vi "Update Set Temp.vi"(8 "error in (no error)":errorcluster, 9 "Setpoint":dbl, 10 "Run":bool, 11 "Test in":refnum<class "Test.lvclass">) -> (0 "error out":errorcluster, 3 "Test out":refnum<class "Test.lvclass">)   [LabVIEW 2019, in "Test.lvlib" / "Test.lvclass"]
uses:
  Test.lvclass
  Test.lvclass/Test.ctl
  <userlib>/_MGI/Application Control/MGI Get Value/MGI Get Value (String).vi
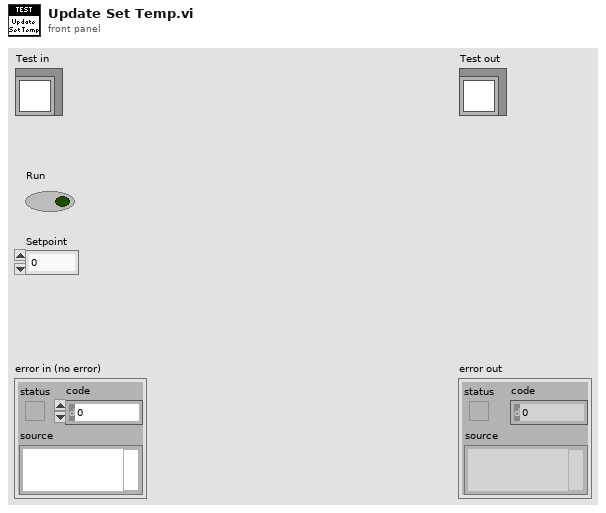
[diagram p1: front panel]
types:
  T1 = map{string, cluster{"Selected Heads":string, "Instrument":refnum<class "Message Enqueuer.lvclass">, "Platform":refnum<class "Message Enqueuer.lvclass">}}
  T2 = typedef "Test.lvlib/Cobra Data.ctl" = cluster{"M2 Dataset":cluster{"Read Temp":dbl, "Feedback":u8, "Set Temp":dbl}, "M1 Dataset":cluster{"Read Temp":dbl, "Feedback":u8, "Set Temp":dbl}, "Comp":bool}
  T3 = cluster{"Selected Heads":string, "Instrument":refnum<class "Message Enqueuer.lvclass">, "Platform":refnum<class "Message Enqueuer.lvclass">}
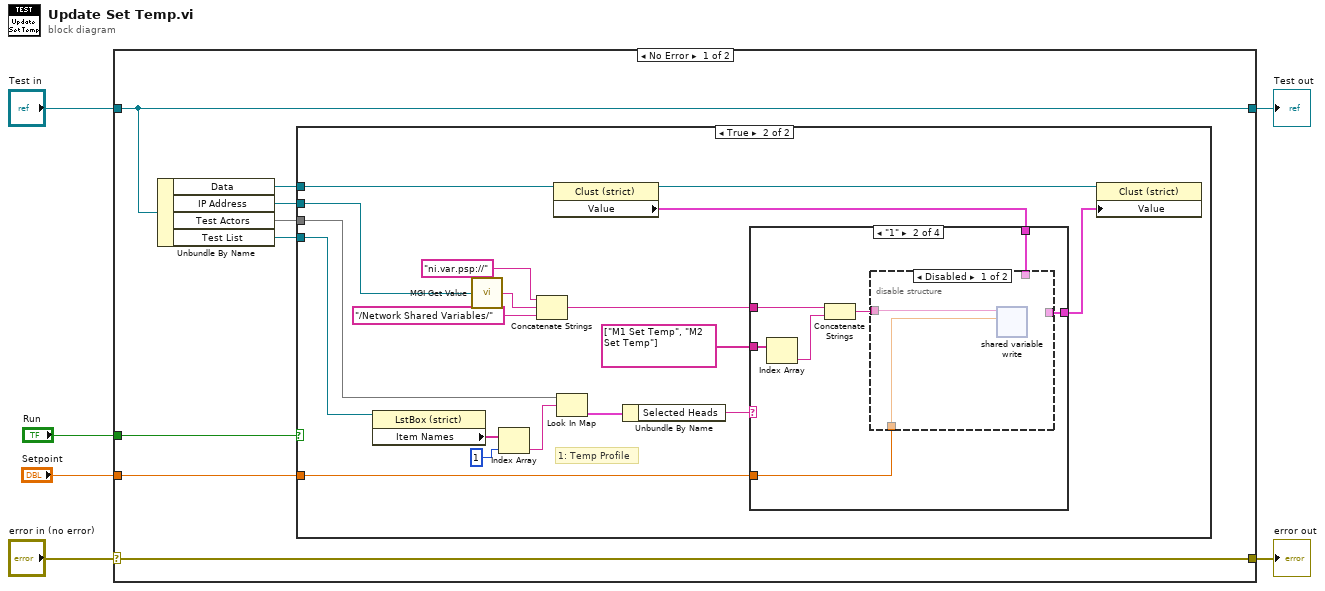
[diagram p0: block diagram]
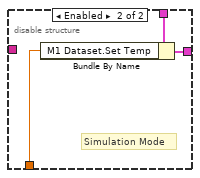
[diagram p4: hidden frame]
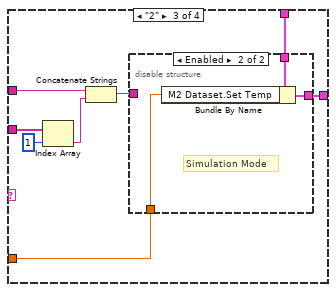
[diagram p5: hidden frame]
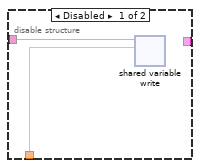
[diagram p6: hidden frame]
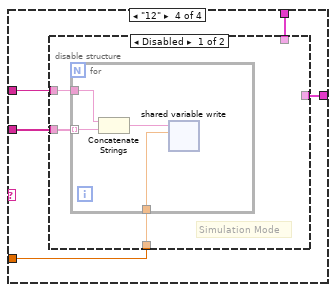
[diagram p7: hidden frame]
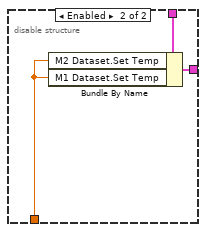
[diagram p8: hidden frame]
diagram:
  n1 = case shown="No Error" "error in (no error)" {
    selector: "error in (no error)" -> [w14 w75]
    tunnel: [w14 w75] -> w5
    tunnel: [w7 w74] -> w3
    tunnel: "Test in" -> [w7 w74]
    tunnel: "Setpoint" -> [w9 _]
    tunnel: "Run" -> [w8 _]
    frame No Error {
      n2 = Unbundle By Name(w7) -> ("Data"=w13:refnum<vi>, "IP Address"=w10:refnum<vi>, "Test Actors"=w11:T1, "Test List"=w12:refnum<vi>)
      n3 = case shown="True" w8 {
        tunnel: w9 -> [_ w32]
        tunnel: w10 -> [_ w22]
        tunnel: w11 -> [_ w29]
        tunnel: w12 -> [_ w28]
        tunnel: w13 -> [_ w18]
        frame False {
        }
        frame True {
          # "1: Temp Profile"
          n4 = property class="LstBox (strict)"(reference=w28) -> ("Item Names"=w31:string[])  [unwired: 1 in, 2 out]
          n5 = call-poly <userlib>:"MGI Get Value.vi"("String Ref"=w22) -> ("String"=w21:string)
          n6 = Index Array(array=w31, index=1) -> (element=w30:string)
          n7 = Concatenate Strings("ni.var.psp://", w21, "/Network Shared Variables/") -> (w23:string)
          n8 = property class="Clust (strict)"(reference=w18) -> (reference out=w17:refnum<vi>, "Value"=w16:T2)  [unwired: 1 in, 1 out]
          n9 = Look In Map(map=w29, key=w30) -> (value=w26:T3)  [unwired: 1 in, 1 out]
          n10 = Unbundle By Name(w26) -> ("Selected Heads"=w25:string)
          n11 = case shown="\"1\"" w25 {
            tunnel: w23 -> [_ w40 w48 w63]
            tunnel: w32 -> [_ w36 w53 w59]
            tunnel: string[] ["M1 Set Temp", "M2 Set Temp"] -> [_ w39 w52 w62]
            tunnel: w16 -> [w33 w35 w50 w61]
            tunnel: [w33 w34 w49 w60] -> w15
            frame "0", Default {
            }
            frame "1" {
              n12 = Index Array(array=w39) -> (element=w38:string)  [unwired: 1 in]
              n13 = Concatenate Strings(w40, w38) -> (w37:string)
              n14 = disable-structure shown="Disabled" {
                disable-tunnel: w36 -> [w42 w43]
                disable-tunnel: w35 -> [_ w45]
                disable-tunnel: [_ w44] -> w34
                disable-tunnel: w37 -> [w41 _]
                frame Disabled {
                  n15 = shared-variable-write(w41, w42) -> ()  [unwired: 1 in, 2 out]
                }
                frame Enabled {
                  # "Simulation Mode"
                  n16 = Bundle By Name(cluster=w45, "M1 Dataset.Set Temp"=w43) -> (w44:T2)
                }
              }
            }
            frame "2" {
              n17 = Index Array(array=w52, index=1) -> (element=w47:string)
              n18 = Concatenate Strings(w48, w47) -> (w46:string)
              n19 = disable-structure shown="Enabled" {
                disable-tunnel: w53 -> [w55 w56]
                disable-tunnel: w50 -> [_ w58]
                disable-tunnel: [_ w57] -> w49
                disable-tunnel: w46 -> [w54 _]
                frame Disabled {
                  n20 = shared-variable-write(w54, w55) -> ()  [unwired: 1 in, 2 out]
                }
                frame Enabled {
                  # "Simulation Mode"
                  n21 = Bundle By Name(cluster=w58, "M2 Dataset.Set Temp"=w56) -> (w57:T2)
                }
              }
            }
            frame "12" {
              n22 = disable-structure shown="Disabled" {
                disable-tunnel: w63 -> [w66 _]
                disable-tunnel: w62 -> [w65 _]
                disable-tunnel: w61 -> [_ w73]
                disable-tunnel: [_ w72] -> w60
                disable-tunnel: w59 -> [w64 w71]
                frame Disabled {
                  # "Simulation Mode"
                  n23 = for {
                    tunnel: w66 -> [w69]
                    tunnel: w65 -> [w68] mode=indexing
                    tunnel: w64 -> [w67]
                    n24 = Concatenate Strings(w69, w68) -> (w70:string)
                    n25 = shared-variable-write(w70, w67) -> ()  [unwired: 1 in, 2 out]
                  }
                }
                frame Enabled {
                  n26 = Bundle By Name(cluster=w73, "M2 Dataset.Set Temp"=w71, "M1 Dataset.Set Temp"=w71) -> (w72:T2)
                }
              }
            }
          }
          n27 = property class="Clust (strict)"(reference=w17, "Value"=w15) -> ()  [unwired: 1 in, 2 out]
        }
      }
    }
    frame Error {
    }
  }
  "error out" <- w5
  "Test out" <- w3
